vi "AK-LNI Antwort empfangen.vi"(8 "Fehler (Eingang)":errorcluster, 11 "VISA resource name":refnum<visa-resource-name>) -> (0 "Fehler (Ausgang)":errorcluster, 1 "ES (Error Status)":string, 2 "Daten":string, 3 "VISA resource name out":refnum<visa-resource-name>, 4 "Lesepuffer":string, 5 "Befehl":string)   [LabVIEW 2020, in "Linearisierung v2.lvlib" / "Gasteiler.lvlib" / "AK Komm Gasteiler.lvlib"]
doc: "Liest die Anwort auf einen AK-Befehl von der COM-Schnittstelle und wertet die Telegrammteile aus:\n\nBefehl: Wiederholung des gesendeten Befehls, Ausnahme ???? ... Befehl unbekannt\nDaten: Daten (String)\nES: Error Status (String), 0..kein Fehler\n\nDer ErrorStatus wird ausgewertet und liefert im Fehlercluster \"Fehler(Ausgang)\" die Fehlerursache in Klartext."
uses:
  AK Komm Gasteiler.lvlib
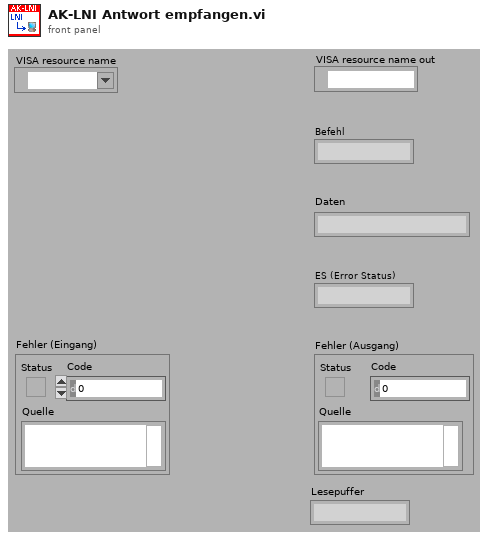
[diagram p1: front panel]
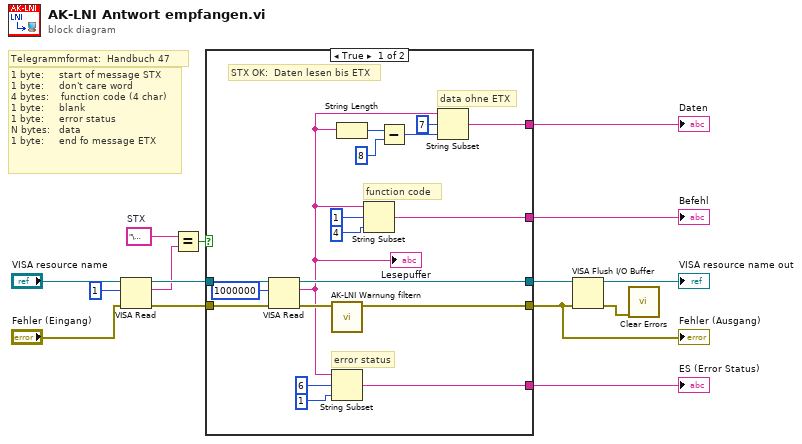
[diagram p0: block diagram]
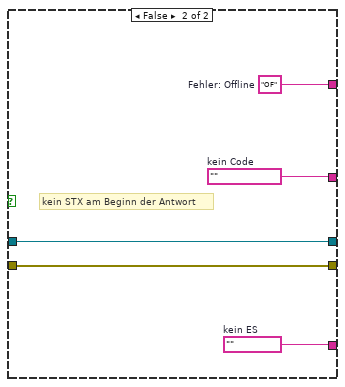
[diagram p2: hidden frame]
diagram:
  w9 = "\u0002"  # STX
  # "Telegrammformat:  Handbuch 47"
  # "1 byte:     start of message STX\n1 byte:     don't care word\n4 bytes:    function code (4 char)\n1 byte:     blank\n1 byte:     error status\nN bytes:   data\n1 byte:     end fo message ETX"
  n1 = VISA Read(VISA resource name="VISA resource name", byte count=u32 1 ("Byte-Anzahl"), error in (no error)="Fehler (Eingang)") -> (VISA resource name out=w11:refnum<visa-resource-name>, read buffer=w4:string, error out=w10:errorcluster)  [unwired: 1 out]
  n2 = Equal?(x=w9, y=w4) -> (x = y?=w5:bool)
  n3 = case shown="True" w5 {
    tunnel: w11 -> [w33 w38]
    tunnel: w10 -> [w32 w37]
    tunnel: [w29 w38] -> w8
    tunnel: [w28 w37] -> w1
    tunnel: [w16 w34] -> w7
    tunnel: [w18 w36] -> w3
    tunnel: [w17 w35] -> w2
    frame True {
      # "error status"
      # "function code"
      # "data ohne ETX"
      # "STX OK:  Daten lesen bis ETX"
      n4 = VISA Read(VISA resource name=w33, byte count=u32 1000000 ("Byte-Anzahl"), error in (no error)=w32) -> (VISA resource name out=w29:refnum<visa-resource-name>, read buffer=w19:string, error out=w30:errorcluster)  [unwired: 1 out]
      "Lesepuffer" <- w19
      n5 = call "AK-LNI Warnung filtern.vi"("error in (no error)"=w30) -> ("error out"=w28:errorcluster)  [unwired: 10 in]
      n6 = String Subset(string=w19, offset (0)=6 ("Offset (0)"), length (rest)=1 ("Länge (Rest)")) -> (substring=w17:string)
      n7 = String Length(string=w19) -> (length=w27:i32)
      n8 = String Subset(string=w19, offset (0)=1 ("Offset (0)"), length (rest)=4 ("Länge (Rest)")) -> (substring=w18:string)
      n9 = Subtract(x=w27, y=8) -> (x-y=w25:i32)
      n10 = String Subset(string=w19, offset (0)=7 ("Offset (0)"), length (rest)=w25) -> (substring=w16:string)
    }
    frame False {
      w34 = "OF"  # Fehler: Offline
      w35 = ""  # kein ES
      w36 = ""  # kein Code
      # "kein STX am Beginn der Antwort"
    }
  }
  "Fehler (Ausgang)" <- w1
  "Daten" <- w7
  "Befehl" <- w3
  "ES (Error Status)" <- w2
  n11 = VISA Flush I/O Buffer(VISA resource name=w8, error in (no error)=w1) -> (VISA resource name out=→"VISA resource name out":refnum<visa-resource-name>, error out=w6:errorcluster)  [unwired: 1 in]
  n12 = call <vilib>:"Clear Errors.vi"("error in (no error)"=w6) -> ()  [unwired: 5 in, 2 out]
